vi "new.vi"(8 "error in":errorcluster, 11 "websocket user plugin in":refnum<class "websocket user plugin.lvclass">) -> (0 "error out":errorcluster, 3 "websocket user plugin out":refnum<class "websocket user plugin.lvclass">)   [LabVIEW 2016, in "websocket user plugin.lvclass"]
uses:
  websocket user plugin.lvclass
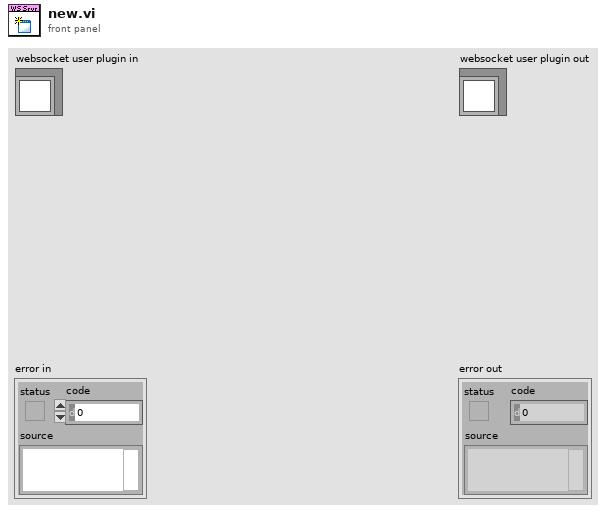
[diagram p1: front panel]
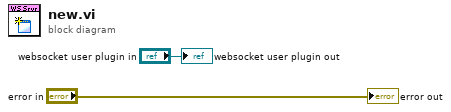
[diagram p0: block diagram]
diagram:
  "error out" <- "error in"
  "websocket user plugin out" <- "websocket user plugin in"
